vi "Workspace.vi"() -> ()   [LabVIEW 2010]
panel:
  in  "Workspace":path
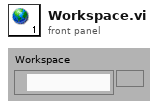
[diagram p1: front panel]
diagram:
